vi "weat.vi"() -> ()   [LabVIEW 2014]
uses:
  subVI/departure.vi
  subVI/Destination.vi
  <vilib>/httpClient/LabVIEWHTTPClient.lvlib
panel:
  out "연결된 문자열":string
  in  "정지":bool
  out "departure":string
  out "Destination":string
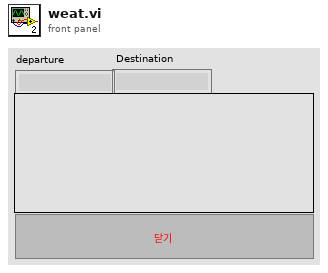
[diagram p1: front panel]
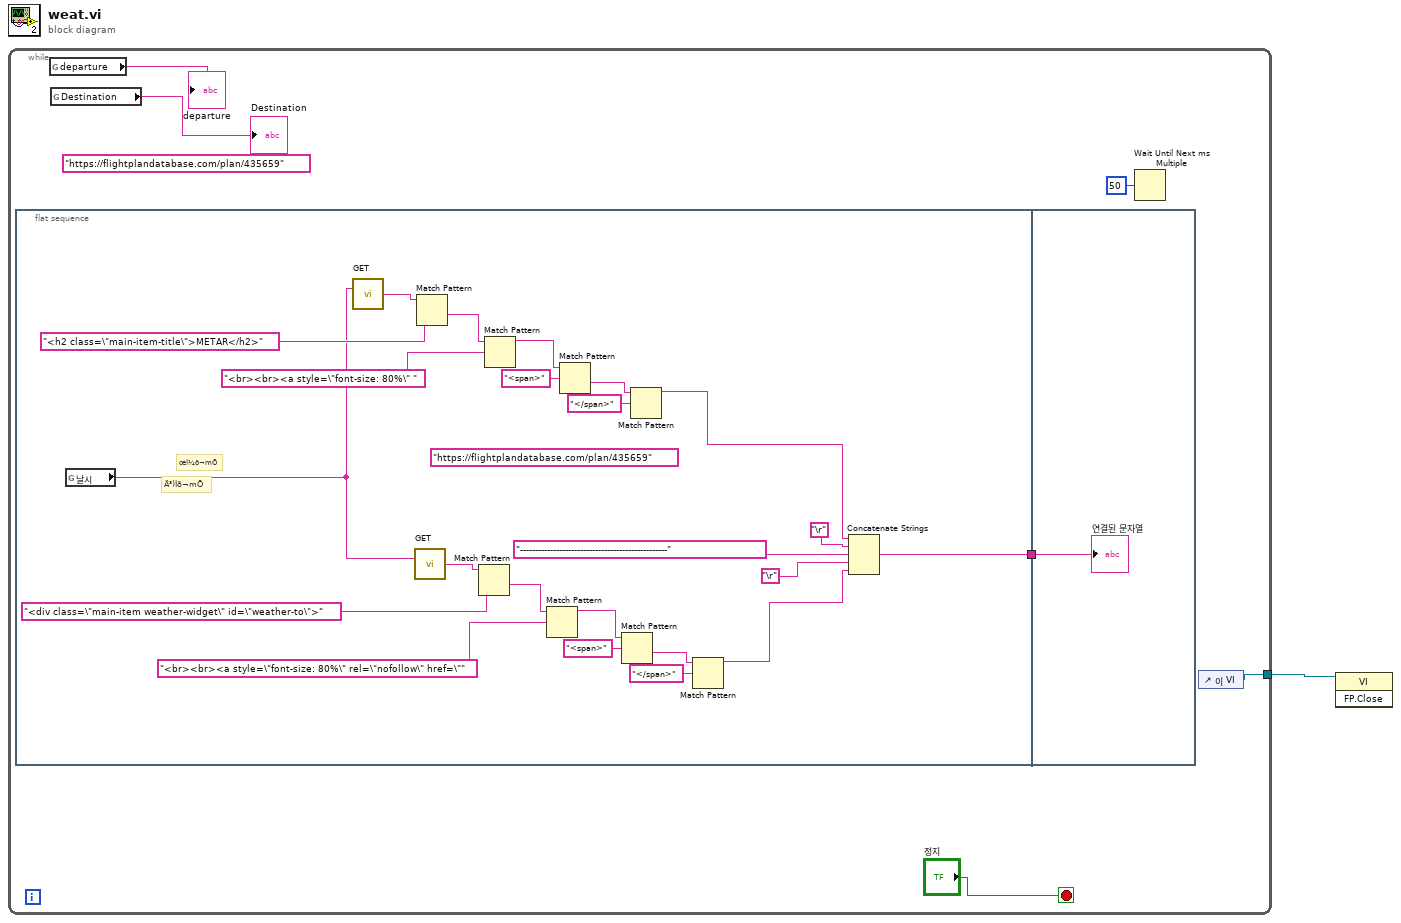
[diagram p0: block diagram]
diagram:
  n1 = while {
    tunnel: [w6] -> w1
    stop <- "정지" stop-if-true
    (unwired) "https://flightplandatabase.com/plan/435659"
    n2 = flat-sequence {
      tunnel: [w8] -> w2
      tunnel: w2 -> [w31]
      frame #0 {
        (unwired) "https://flightplandatabase.com/plan/435659"
        # "œÍ¼õ¬mÕ"
        # "Ä³)Ìõ¬mÕ"
        n3 = global read "날시.vi" "날시"() -> (w14:string)
        n4 = call <vilib>:"GET.vi"("url"=w14) -> ("body"=w30:string)  [unwired: 11 in, 3 out]
        n5 = call <vilib>:"GET.vi"("url"=w14) -> ("body"=w15:string)  [unwired: 11 in, 3 out]
        n6 = Match Pattern(string=w30, regular expression="<h2 class=\"main-item-title\">METAR</h2>" ("정규식")) -> (after substring=w28:string)  [unwired: 1 in, 3 out]
        n7 = Match Pattern(string=w15, regular expression="<div class=\"main-item weather-widget\" id=\"weather-to\">" ("정규식")) -> (after substring=w17:string)  [unwired: 1 in, 3 out]
        n8 = Match Pattern(string=w28, regular expression="<br><br><a style=\"font-size: 80%\" " ("정규식")) -> (before substring=w26:string)  [unwired: 1 in, 3 out]
        n9 = Match Pattern(string=w17, regular expression="<br><br><a style=\"font-size: 80%\" rel=\"nofollow\" href=\"" ("정규식")) -> (before substring=w19:string)  [unwired: 1 in, 3 out]
        n10 = Match Pattern(string=w26, regular expression="<span>" ("정규식")) -> (after substring=w24:string)  [unwired: 1 in, 3 out]
        n11 = Match Pattern(string=w19, regular expression="<span>" ("정규식")) -> (after substring=w21:string)  [unwired: 1 in, 3 out]
        n12 = Match Pattern(string=w24, regular expression="</span>" ("정규식")) -> (before substring=w10:string)  [unwired: 1 in, 3 out]
        n13 = Match Pattern(string=w21, regular expression="</span>" ("정규식")) -> (before substring=w11:string)  [unwired: 1 in, 3 out]
        n14 = Concatenate Strings(w10, "\r", "-------------------------------------------------" ("문자열"), "\r", w11) -> (w8:string)
      }
      frame #1 {
        "연결된 문자열" <- w31
      }
    }
    n15 = global read "departure.vi" "departure"() -> (→"departure":string)
    n16 = global read "Destination.vi" "Destination"() -> (→"Destination":string)
    n17 = Wait Until Next ms Multiple(millisecond multiple=u32 50 ("ms 배수")) -> ()  [unwired: 1 out]
    n18 = control-ref of="이 VI"() -> (w6:refnum<vi>)
  }
  n19 = invoke class="VI" method="FP.Close"(reference=w1) -> ()  [unwired: 2 in, 3 out]
